vi "Quadratic Roots.vi"() -> ()   [LabVIEW 2024]
panel:
  out "Root 2":dbl
  out "Root1":dbl
  in  "C":dbl
  in  "B":dbl
  in  "A":dbl
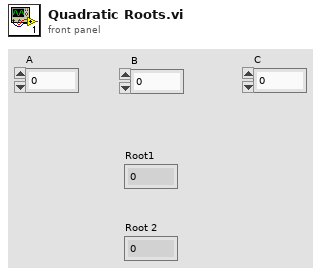
[diagram p1: front panel]
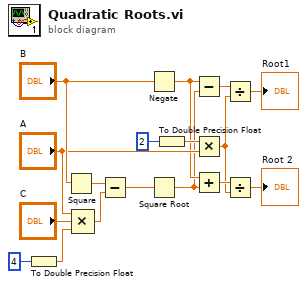
[diagram p0: block diagram]
diagram:
  n1 = To Double Precision Float(number=4) -> (double precision float=w10:dbl)
  n2 = Square(x="B") -> (x^2=w14:dbl)
  n3 = Compound Arithmetic op=MULTIPLY("A", "C", w10) -> (w9:dbl)
  n4 = Subtract(x=w14, y=w9) -> (x-y=w8:dbl)
  n5 = Negate(x="B") -> (-x=w5:dbl)
  n6 = Square Root(x=w8) -> (sqrt(x)=w4:dbl)
  n7 = To Double Precision Float(number=2) -> (double precision float=w16:dbl)
  n8 = Subtract(x=w5, y=w4) -> (x-y=w7:dbl)
  n9 = Multiply(x=w16, y="A") -> (x*y=w2:dbl)
  n10 = Add(x=w5, y=w4) -> (x+y=w3:dbl)
  n11 = Divide(x=w7, y=w2) -> (x/y=→"Root1":dbl)
  n12 = Divide(x=w3, y=w2) -> (x/y=→"Root 2":dbl)
